vi "H036 Harsh Pandit SCADA Lab 4c Sem 6.vi"() -> ()   [LabVIEW 2018]
panel:
  in  "Amplitude":dbl(knob) scale=0.0..10.0
  in  "Frequency":dbl(knob) scale=0.0..10.0
  out "Waveform Chart 2":dbl(graph)
  # "Experiment 4c: Develope sine wave generator using While loop. Vary the amplitude and frequency using knob"
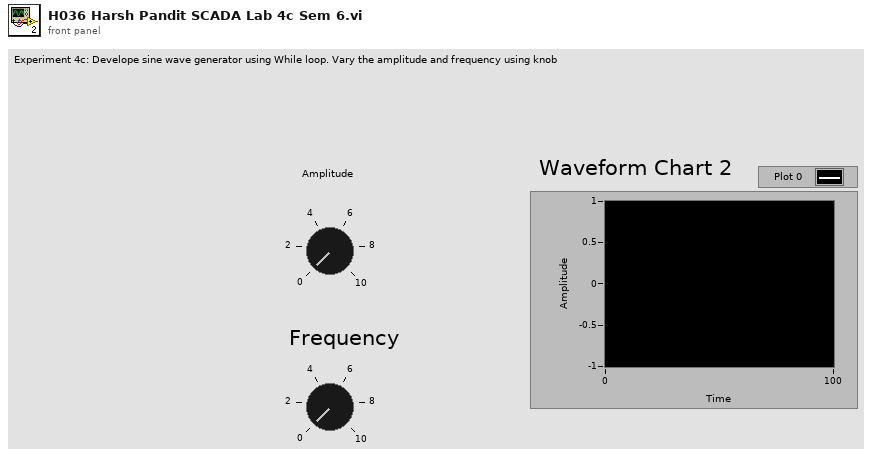
[diagram p1: front panel]
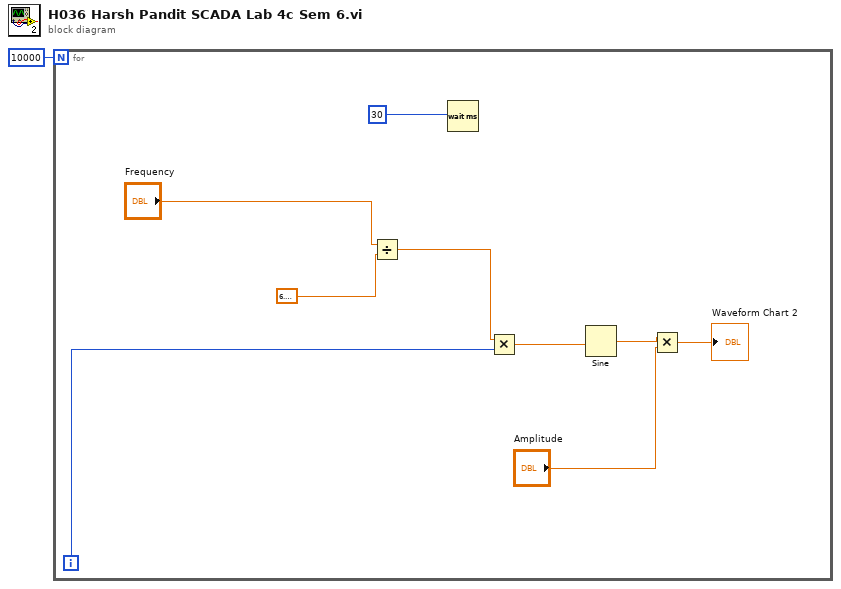
[diagram p0: block diagram]
diagram:
  n1 = for {
    N: 10000 -> [_]
    i -> [w2]
    n2 = Divide(x="Frequency", y=6.283185307179586) -> (x/y=w8:dbl)
    n3 = Wait (ms)(milliseconds to wait=30) -> ()  [unwired: 1 out]
    n4 = Multiply(x=w8, y=w2) -> (x*y=w7:dbl)
    n5 = Sine(x=w7) -> (sin(x)=w6:dbl)
    n6 = Multiply(x=w6, y="Amplitude") -> (x*y=→"Waveform Chart 2":dbl)
  }
